vi "S2C_FORNAX_Poly_InstrumentSettingCommand.vi"(8 "Error In":errorcluster, 10 "InstrumentSettingCommand":T4={"Partition"="Default", "Message"="InstrumentSettingCommand", "M_EnergyChannelId"=0, "M_InstrumentType"=0, "M_SettingType"=0, "M_SettingValue"=0} {"M_SettingType" items=["CUT_SWITCH_ENABLE_SETTING"=0, "LIGASURE_HANDSWITCH_ENABLE_SETTING"=1, "SHARED_COAG_IN_USE_SETTING"=2, "AUTOBIPOLAR_IN_USE_SETTING"=3, "AMMETER_IN_USE_SETTING"=4, "ENDO_IN_USE_SETTING"=5, "SETTING_TYPE_NOT_USED"=-1]; "M_InstrumentType" items=["INSTRUMENT_TYPE_UNKNOWN", "INSTRUMENT_TYPE_MONOPOLAR", "INSTRUMENT_TYPE_BIPOLAR", "INSTRUMENT_TYPE_TRIVERSE", "INSTRUMENT_TYPE_LIGASURE", "INSTRUMENT_TYPE_ADVANCE_II", "INSTRUMENT_TYPE_BIPOLAR_RESECTION", "INSTRUMENT_TYPE_HOOK", "INSTRUMENT_TYPE_BIZACT", "INSTRUMENT_TYPE_CARDIOBLATE_BIP", "INSTRUMENT_TYPE_CARDIOBLATE_BIP_GEMINI_S", "INSTRUMENT_TYPE_CARDIOBLATE_MONO", "INSTRUMENT_TYPE_ULTRASONIC", "INSTRUMENT_TYPE_MONOPOLAR_GI", "INSTRUMENT_TYPE_GOLDILOCKS"]; "M_EnergyChannelId" items=["EC_MONO_1"=0, "EC_BIPOLAR"=1, "EC_MONO_2"=2, "EC_ADVANCED"=3, "EC_ADVANCED_ECUT"=4, "EC_ADVANCED_DCUT"=5, "EC_SHARED_COAG"=6, "EC_INTERNAL_BIP_CAL"=7, "EC_NOT_USED"=-1]}, 11 "Settings":T5={"Driver"="Fornax", "Command"="InstrumentSettingCommand", "Return"="ErrorStatus", "Parameters"="", "Timeout"=10.0}) -> (0 "Error Out":errorcluster, 3 "Response":string)   [LabVIEW 2015]
uses:
  Typedefs/EnergyChannelId.ctl
  Typedefs/InstrumentType.ctl
  Typedefs/InstrumentSettingType.ctl
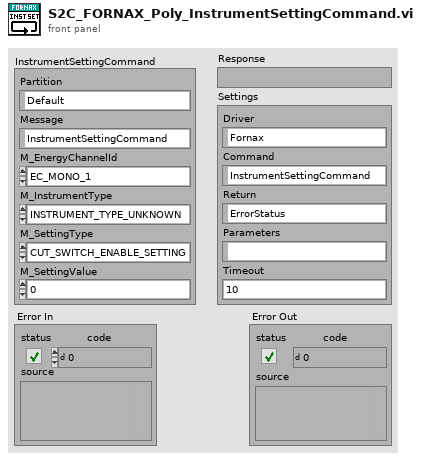
[diagram p1: front panel]
types:
  T1 = typedef "EnergyChannelId.ctl" = i16
  T2 = typedef "InstrumentType.ctl" = i16
  T3 = typedef "InstrumentSettingType.ctl" = i16
  T4 = cluster{"Partition":string, "Message":string, "M_EnergyChannelId":T1, "M_InstrumentType":T2, "M_SettingType":T3, "M_SettingValue":i32}
  T5 = cluster{"Driver":string, "Command":string, "Return":string, "Parameters":string, "Timeout":dbl}
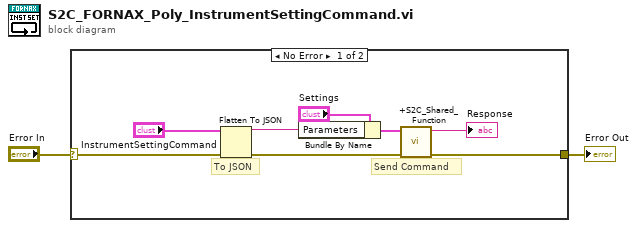
[diagram p0: block diagram]
diagram:
  n1 = case shown="No Error" "Error In" {
    selector: "Error In" -> [w6 w11]
    tunnel: [w5 w11] -> w1
    frame No Error {
      # "To JSON"
      # "Send Command"
      n2 = Flatten To JSON(anything="InstrumentSettingCommand", error in (no error)=w6) -> (JSON string=w7:string, 11:w9:errorcluster)  [unwired: 1 in]
      n3 = Bundle By Name(cluster="Settings", "Parameters"=w7) -> (w10:T5)
      n4 = call "+S2C_Shared_Function.vi"("Error In"=w9, "Settings"=w10) -> ("Error Out"=w5:errorcluster, "Response"=→"Response":string)  [unwired: 8 in]
    }
    frame Error {
    }
  }
  "Error Out" <- w1
